vi "Ramp (G3)-Create.vi"(0 "Ramp in":T1, 5 "Sampling Rate (Hz)":dbl, 7 "Npts":i32, 9 "RepNum":i32, 11 "error in (no error)":errorcluster) -> (4 "Ramp out":T1, 6 "Waveform":dbl[](array[numeric]), 15 "error out":errorcluster)   [LabVIEW 2020]
uses:
  Ramp.Properties.ctl
  <vilib>/Analysis/1siggen.llb/Ramp Pattern by Samples.vi
  <vilib>/Analysis/NI_AALBase.lvlib
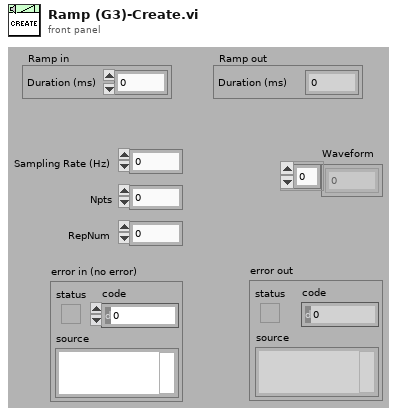
[diagram p1: front panel]
types:
  T1 = typedef "Ramp.Properties.ctl" = cluster{"Duration (ms)":dbl}
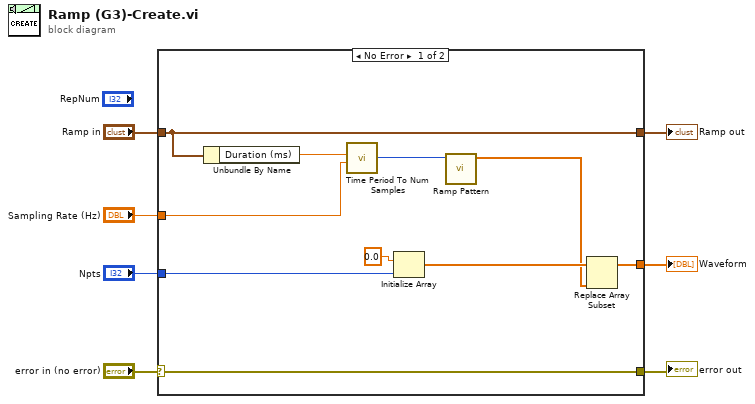
[diagram p0: block diagram]
diagram:
  n1 = case shown="No Error" "error in (no error)" {
    selector: "error in (no error)" -> [w17 w19]
    tunnel: [w17 w19] -> w6
    tunnel: [w16 w18] -> w4
    tunnel: "Ramp in" -> [w16 w18]
    tunnel: "Npts" -> [w13 _]
    tunnel: "Sampling Rate (Hz)" -> [w12 _]
    tunnel: [w8 _] -> w1
    frame No Error {
      n2 = Unbundle By Name(w16) -> ("Duration (ms)"=w15:dbl)
      n3 = call "Time Period To Num Samples.vi"("Duration (ms)"=w15, "Sampling rate (Hz)"=w12) -> ("Samples"=w14:i32)  [unwired: 5 in]
      n4 = Initialize Array(0.0, w13) -> (w10:dbl[])
      n5 = call-poly <vilib>:"Ramp Pattern.vi"("samples"=w14) -> ("Ramp Pattern"=w9:dbl[])  [unwired: 9 in, 1 out]
      n6 = Replace Array Subset(array=w10, new element=w9) -> (w8:dbl[])  [unwired: 1 in]
    }
    frame Error {
    }
  }
  "error out" <- w6
  "Ramp out" <- w4
  "Waveform" <- w1
